vi "scan2d_perform_raster_scan.vi"(8 "error in (no error)":errorcluster, 11 "scan_2d in":refnum<class "scan_2d.lvclass">) -> (0 "error out":errorcluster, 3 "scan_2d out":refnum<class "scan_2d.lvclass">)   [LabVIEW 2015, in "scan_2d.lvclass"]
uses:
  scan_2d.lvclass
  scan_2d.lvclass/scan_2d.ctl
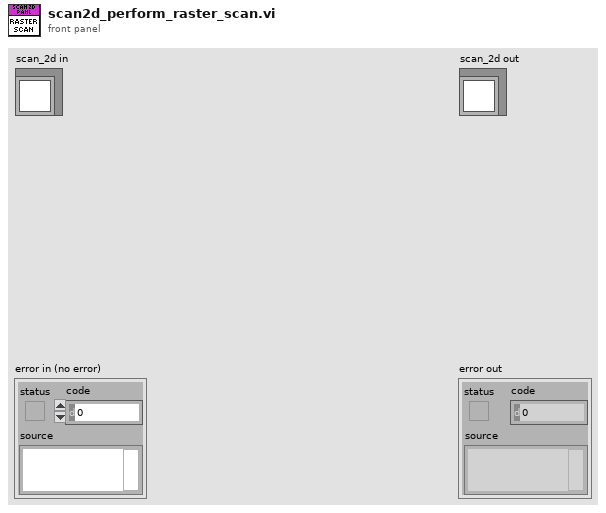
[diagram p1: front panel]
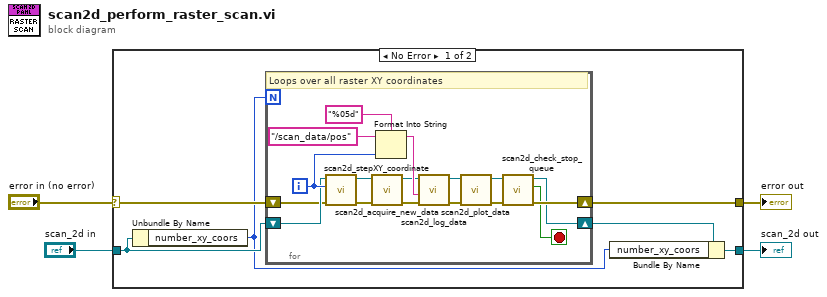
[diagram p0: block diagram]
diagram:
  n1 = case shown="No Error" "error in (no error)" {
    selector: "error in (no error)" -> [w10 w29]
    tunnel: [w8 w29] -> w3
    tunnel: [w9 w28] -> w1
    tunnel: "scan_2d in" -> [w7 w28]
    frame No Error {
      n2 = Unbundle By Name(w7) -> ("number_xy_coors"=w5:i32)
      n3 = for {
        N: w5 -> [_]
        shift-right: [w24] -> w8
        shift-left: w10 -> [w11]
        shift-right: [w22] -> w6
        shift-left: w7 -> [w17]
        i -> [w18]
        stop <- w16 stop-if-true
        # "Loops over all raster XY coordinates"
        n4 = call "scan2d_stepXY_coordinate.vi"("error in (no error)"=w11, "Step#"=w18, "scan_2d in"=w17) -> ("error out"=w12:errorcluster, "scan_2d out"=w15:refnum<class "scan_2d.lvclass">)  [unwired: 7 in]
        n5 = call "scan2d_acquire_new_data.vi"("error in (no error)"=w12, "scan_2d in"=w15) -> ("error out"=w13:errorcluster, "scan_2d out"=w14:refnum<class "scan_2d.lvclass">)  [unwired: 8 in]
        n6 = Format Into String(format string="%05d", initial string="/scan_data/pos", w18) -> (resulting string=w19:string)  [unwired: 1 in, 1 out]
        n7 = call "scan2d_log_data.vi"("error in (no error)"=w13, "location"=w19, "scan_2d in"=w14) -> ("error out"=w21:errorcluster, "scan_2d out"=w20:refnum<class "scan_2d.lvclass">)  [unwired: 7 in]
        n8 = call "scan2d_plot_data.vi"("error in (no error)"=w21, "scan_panel in"=w20) -> ("error out"=w25:errorcluster, "scan_panel out"=w23:refnum<class "scan_2d.lvclass">)  [unwired: 8 in]
        n9 = call "scan2d_check_stop_queue.vi"("error in (no error)"=w25, "scan_panel in"=w23) -> ("error out"=w24:errorcluster, "stop?"=w16:bool, "scan_panel out"=w22:refnum<class "scan_2d.lvclass">)  [unwired: 7 in]
      }
      n10 = Bundle By Name(cluster=w6, "number_xy_coors"=w5) -> (w9:refnum<class "scan_2d.lvclass">)
    }
    frame Error {
    }
  }
  "error out" <- w3
  "scan_2d out" <- w1
